vi "select_user.vi"(6 "user":refnum<vi>, 8 "error in":errorcluster) -> (0 "error out":errorcluster)   [LabVIEW 2010]
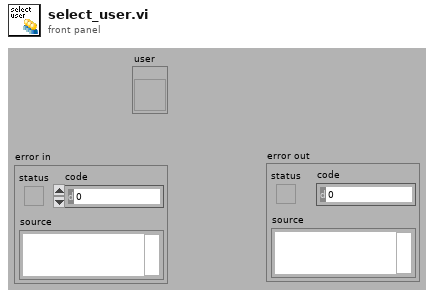
[diagram p1: front panel]
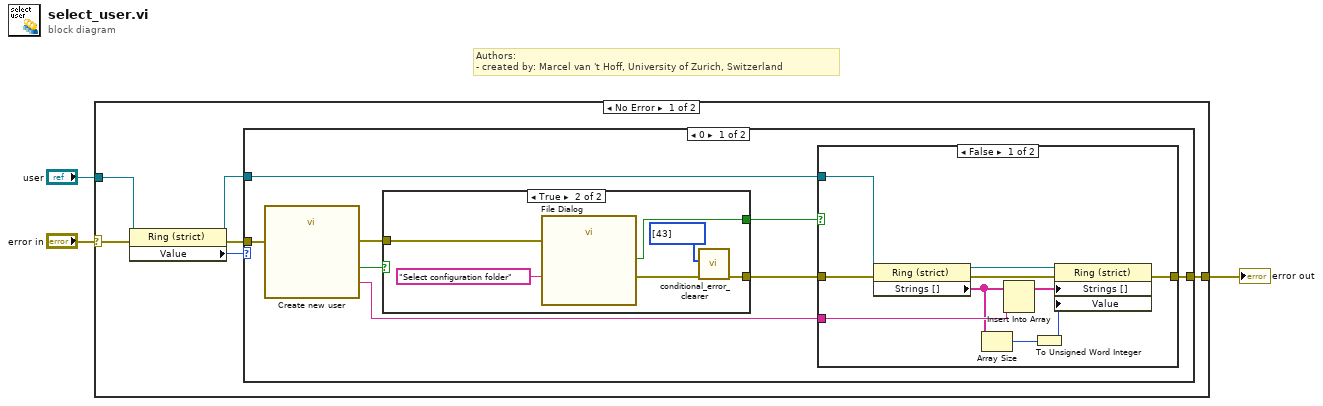
[diagram p0: block diagram]
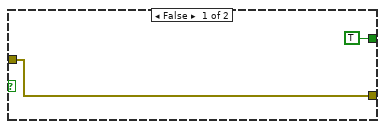
[diagram p2: hidden frame]
diagram:
  # "Authors: \n- created by: Marcel van 't Hoff, University of Zurich, Switzerland"
  n1 = case shown="No Error" "error in" {
    selector: "error in" -> [w7 w38]
    tunnel: [w8 w38] -> w2
    tunnel: "user" -> [w9 _]
    frame No Error {
      n2 = property class="Ring (strict)"(reference=w9, error in=w7) -> (reference out=w4:refnum<vi>, error out=w6:errorcluster, "Value"=w5:u16)
      n3 = case shown="0" w5 {
        tunnel: w6 -> [w17 w37]
        tunnel: [w15 w37] -> w8
        tunnel: w4 -> [w14 _]
        frame 0 {
          n4 = call "Create new user"("error in (no error)"=w17) -> ("Name:"=w16:string, "OK"=w13:bool, "error out"=w12:errorcluster)  [unwired: 16 in]
          n5 = case shown="True" w13 {
            tunnel: w12 -> [w19 w23]
            tunnel: [w19 w22] -> w11
            tunnel: [TRUE ("cancelled") w21] -> w10
            frame False {
            }
            frame True {
              n6 = call "File Dialog"("prompt"="Select configuration folder", "error in"=w23) -> ("cancelled"=w21:bool, "error out"=w24:errorcluster)  [unwired: 10 in, 2 out]
              n7 = call "conditional_error_clearer.vi"("error in (no error)"=w24, "array of clearable error codes"=i32[] [43]) -> ("error out"=w22:errorcluster)  [unwired: 9 in]
            }
          }
          n8 = case shown="False" w10 {
            tunnel: w16 -> [w31 _]
            tunnel: [w27 w36] -> w15
            tunnel: w11 -> [w26 w36]
            tunnel: w14 -> [w35 _]
            frame False {
              n9 = property class="Ring (strict)"(reference=w35, error in=w26) -> (reference out=w32:refnum<vi>, error out=w34:errorcluster, "Strings []"=w30:string[])
              n10 = Array Size(array=w30) -> (size(s)=w29:i32)
              n11 = Insert Into Array(array=w30, new element=w31) -> (w33:string[])  [unwired: 1 in]
              n12 = To Unsigned Word Integer(number=w29) -> (unsigned 16bit integer=w28:u16)
              n13 = property class="Ring (strict)"(reference=w32, error in=w34, "Strings []"=w33, "Value"=w28) -> (error out=w27:errorcluster)  [unwired: 1 out]
            }
            frame True {
            }
          }
        }
        frame Default {
        }
      }
    }
    frame Error {
    }
  }
  "error out" <- w2
